vi "Unflatten.vi"(8 "error in (no error)":errorcluster, 10 "JSON stream":string, 11 "JSON Scalar in":refnum<class "JSON Scalar.lvclass">) -> (0 "error out":errorcluster, 1 "Empty?":bool, 2 "rest of JSON stream":string, 3 "JSON Scalar out":refnum<class "JSON Scalar.lvclass">)   [LabVIEW 2020, in "Library Commun.lvlib" / "JSON Scalar.lvclass"]
uses:
  JSON Scalar.lvclass
  <vilib>/Utility/error.llb/whitespace.ctl
  JSON Scalar.lvclass/JSON Scalar.ctl
  JSON Value/JSON Value.lvclass
  <vilib>/regexp/Match Regular Expression.xnode
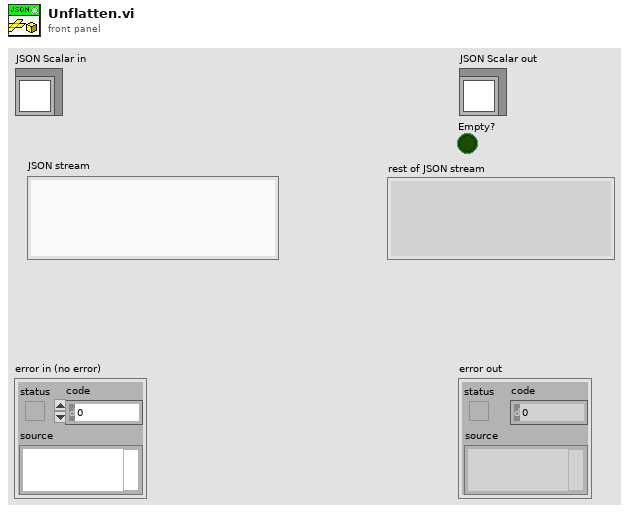
[diagram p1: front panel]
types:
  T1 = typedef "whitespace.ctl" = u16
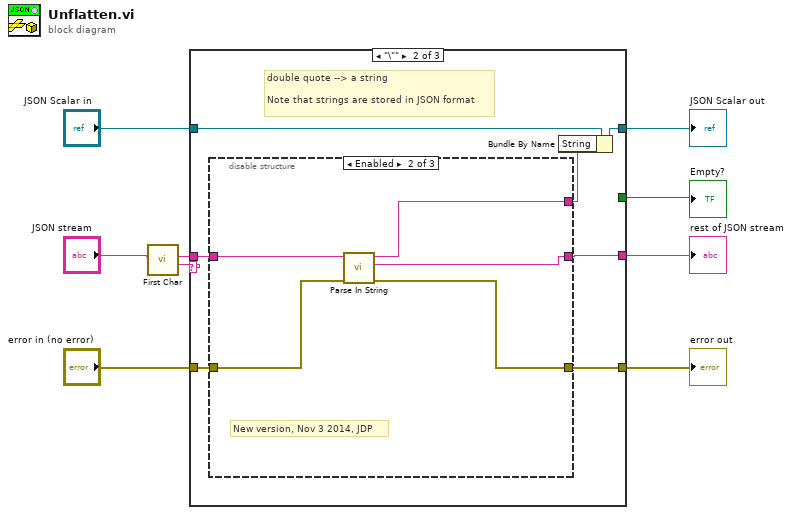
[diagram p0: block diagram]
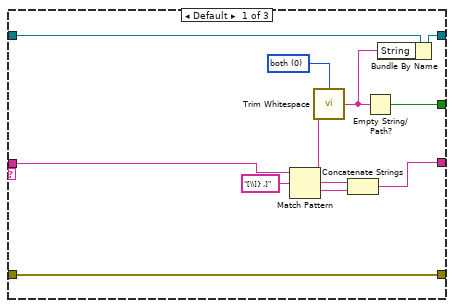
[diagram p2: hidden frame]
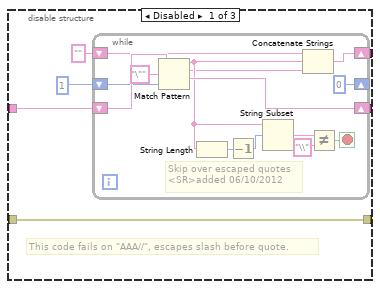
[diagram p3: hidden frame]
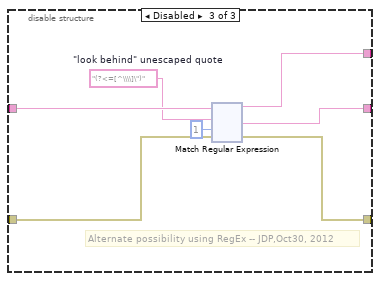
[diagram p4: hidden frame]
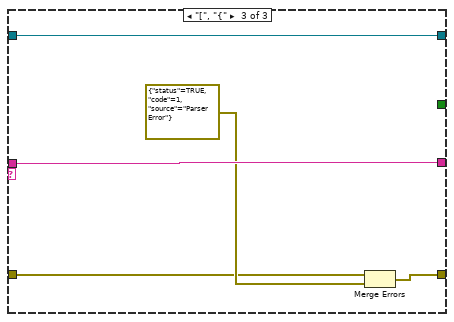
[diagram p5: hidden frame]
diagram:
  n1 = call "First Char.vi"("String in"="JSON stream") -> ("First Char"=w4:string, "String"=w5:string)  [unwired: 9 in]
  n2 = case shown="\"\\\"\"" w4 {
    tunnel: "error in (no error)" -> [w21 w23 w172]
    tunnel: [w21 w22 w175] -> w8
    tunnel: w5 -> [w20 w24 w176]
    tunnel: [w17 w27 w174] -> w7
    tunnel: "JSON Scalar in" -> [w18 w28 w174]
    tunnel: [w14 w25 w176] -> w2
    tunnel: [w10 _ _] -> w1
    frame Default {
      w13 = T1 0 items=["both", "start of string", "end of string"] ("location (both)")
      n3 = Match Pattern(string=w20, regular expression="[\\]} ,]") -> (before substring=w12:string, match substring=w16:string, after substring=w15:string)  [unwired: 1 in, 1 out]
      n4 = call <vilib>:"Trim Whitespace.vi"("string"=w12, "location (both)"=w13) -> ("trimmed string"=w11:string)
      n5 = Concatenate Strings(w16, w15) -> (w14:string)
      n6 = Empty String/Path?(string/path=w11) -> (empty?=w10:bool)
      n7 = Bundle By Name(cluster=w18, "String"=w11) -> (w17:refnum<class "JSON Scalar.lvclass">)
    }
    frame "\"" {
      # "double quote --> a string\n\nNote that strings are stored in JSON format"
      n8 = disable-structure shown="Enabled" {
        disable-tunnel: [w33 w51 w59] -> w26
        disable-tunnel: [w32 w53 w58] -> w25
        disable-tunnel: w24 -> [w29 w52 w60]
        disable-tunnel: w23 -> [w31 w50 w56]
        disable-tunnel: [w31 w49 w55] -> w22
        frame Disabled {
          # "This code fails on \"AAA//\", escapes slash before quote."
          n9 = while {
            shift-right: [w45] -> w33
            shift-left: "" -> [w38]
            shift-right: [w44] -> w32
            shift-left: w29 -> [w43]
            shift-right: [0 ("offset (0)")] -> _
            shift-left: 1 ("offset (0)") -> [w36]
            stop <- w46 stop-if-true
            # "Skip over escaped quotes\n<SR>added 06/10/2012"
            n10 = Match Pattern(string=w43, regular expression="\"", offset (0)=w36) -> (before substring=w42:string, match substring=w37:string, after substring=w44:string)  [unwired: 1 out]
            n11 = String Length(string=w42) -> (length=w41:i32)
            n12 = Decrement(x=w41) -> (x-1=w40:i32)
            n13 = String Subset(string=w42, offset (0)=w40) -> (substring=w39:string)  [unwired: 1 in]
            n14 = Concatenate Strings(w38, w42, w37) -> (w45:string)
            n15 = Not Equal?(x=w39, y="\\") -> (x != y?=w46:bool)
          }
        }
        frame Enabled {
          # "New version, Nov 3 2014, JDP"
          n16 = call "Parse In String.vi"("error in (no error)"=w50, "Partial JSON (starting with quote)"=w52) -> ("error out"=w49:errorcluster, "Rest of JSON"=w53:string, "String (incl quotes)"=w51:string)  [unwired: 7 in]
        }
        frame Disabled {
          w57 = "(?<=[^\\\\]\")"  # "look behind" unescaped quote
          # "Alternate possibility using RegEx -- JDP,Oct30, 2012"
          n17 = xnode "Match Regular Expression"("input string"=w60, "regular expression"=w57, "offset (0)"=1, "error in"=w56) -> ("before match"=w59:string, "after match"=w58:string, "error out"=w55:errorcluster)  [unwired: 2 in, 2 out]
        }
      }
      n18 = Bundle By Name(cluster=w28, "String"=w26) -> (w27:refnum<class "JSON Scalar.lvclass">)
    }
    frame "[", "{" {
      n19 = Merge Errors(w172, errorcluster {"status"=TRUE, "code"=1, "source"="Parser Error"} ("error in")) -> (w175:errorcluster)
    }
  }
  "error out" <- w8
  "JSON Scalar out" <- w7
  "rest of JSON stream" <- w2
  "Empty?" <- w1
